vi "Set Bitmap.vi"(8 "error in (no error)":errorcluster, 10 "Bitmap":u32[][](array[numeric]), 11 "VI Icon Canvas in":refnum<class "VI Icon Canvas.lvclass">) -> (0 "error out":errorcluster, 3 "VI Icon Canvas out":refnum<class "VI Icon Canvas.lvclass">)   [LabVIEW 2023, in "Font Glyph Drawer Interface.lvlib" / "VI Icon Canvas.lvclass"]
uses:
  VI Icon Canvas.lvclass
  VI Icon Canvas.lvclass/VI Icon Canvas.ctl
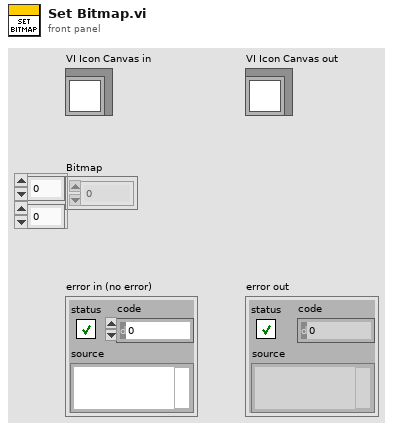
[diagram p1: front panel]
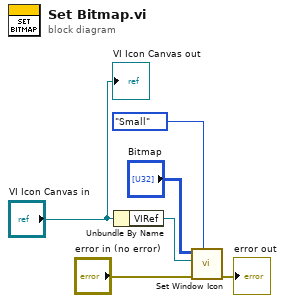
[diagram p0: block diagram]
diagram:
  n1 = Unbundle By Name("VI Icon Canvas in") -> ("VIRef"=w4:refnum<vi>)
  n2 = call "Set Window Icon.vi"("Icon Type"=enum32{"Small", "Big"}."Small", "error in (no error)"="error in (no error)", "VIRef (calling VI)"=w4, "RGB Image"="Bitmap") -> ("Error Out"=→"error out":errorcluster)  [unwired: 7 in]
  "VI Icon Canvas out" <- "VI Icon Canvas in"
